vi "SendCommand.vi"(8 "error in (no error)":errorcluster, 10 "Command string":string, 11 "InstControl in":refnum<class "InstrControl.lvclass">) -> (0 "error out":errorcluster, 3 "InstControl out":refnum<class "InstrControl.lvclass">)   [LabVIEW 2018, in "InstrControl.lvclass"]
uses:
  InstrControl.lvclass
  InstrControl.lvclass/InstrControl.ctl
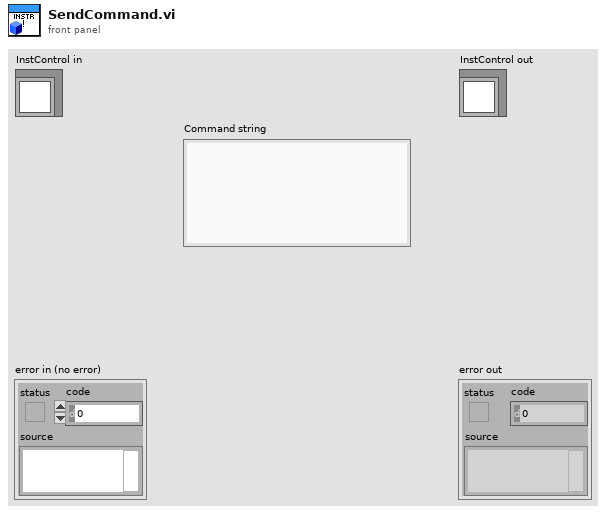
[diagram p1: front panel]
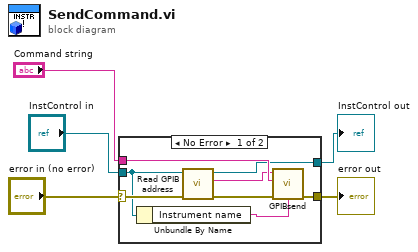
[diagram p0: block diagram]
diagram:
  n1 = case shown="No Error" "error in (no error)" {
    selector: "error in (no error)" -> [w9 w15]
    tunnel: [w13 w15] -> w4
    tunnel: [w10 w14] -> w3
    tunnel: "InstControl in" -> [w7 w14]
    tunnel: "Command string" -> [w12 _]
    frame No Error {
      n2 = Unbundle By Name(w7) -> ("Instrument name"=w6:string)
      n3 = call-dynamic "Read GPIB address.vi"("error in (no error)"=w9, "InstControl in"=w7) -> ("error out"=w8:errorcluster, "GPIB address"=w11:string, "InstControl out"=w10:refnum<class "InstrControl.lvclass">)  [unwired: 7 in]
      n4 = call "GPIBsend.vi"("address string"=w11, "write buffer"=w12, "source"=w6, "error in"=w8) -> ("error out"=w13:errorcluster)  [unwired: 3 in, 2 out]
    }
    frame Error {
    }
  }
  "error out" <- w4
  "InstControl out" <- w3
